vi "bin multiple xy graphs-b.vi"(2 "Error Bar Type":T1(ring), 3 "interval":dbl, 4 "FIXED X INTERVAL?":bool, 5 "parameter 2,3,4 vs 1":cluster{"y vector":dbl[], "avg optspec":dbl[]}[](graph)=[{"y vector"=array[1339 elements], "avg optspec"=array[1339 elements]}, {"y vector"=array[1339 elements], "avg optspec"=array[1339 elements]}, {"y vector"=array[1339 elements], "avg optspec"=array[1339 elements]}]) -> (0 "avgs and errors":dbl[][](array[numeric]), 1 "Array":cluster{"y vector":dbl[], "avg optspec":dbl[]}[](array[cluster]))   [LabVIEW 2009]
panel:
  out "xy graph":cluster{dbl[], dbl[]}[](graph)=[{[5.5, 15.5, 25.5, 35.5, 45.5, 55.5, 0.0], [0.1, 0.1, 0.15, 0.15, 0.2, 0.2, 0.0]}, {[5.5, 5.5, nan, 15.5, 15.5, nan, 25.5, 25.5, nan, 35.5, 35.5, nan, 45.5, 45.5, nan, 55.5, 55.5, nan, 0.0, 0.0, nan], [0.1, 0.1, nan, 0.1, 0.1, nan, 0.15, 0.15, nan, 0.15, 0.15, nan, 0.2, 0.2, nan, 0.2, 0.2, nan, 0.0, 0.0, nan]}, {[5.5, 15.5, 25.5, 35.5, 45.5, 55.5, 0.0], [5.5, 15.5, 25.5, 35.5, 45.5, 55.5, 0.0]}, {[5.5, 5.5, nan, 15.5, 15.5, nan, 25.5, 25.5, nan, 35.5, 35.5, nan, 45.5, 45.5, nan, 55.5, 55.5, nan, 0.0, 0.0, nan], [3.0, 8.0, nan, 13.0, 18.0, nan, 23.0, 28.0, nan, 33.0, 38.0, nan, 43.0, 48.0, nan, 53.0, 58.0, nan, 0.0, 0.0, nan]}]
  out "Array avgs and errors":dbl[][][](array[numeric])
  out "parameter 2,3,4 vs 2":cluster{"y vector":dbl[], "avg optspec":dbl[]}(graph)
  # "avgx\navgy\nerrorlow\nerrorhigh"
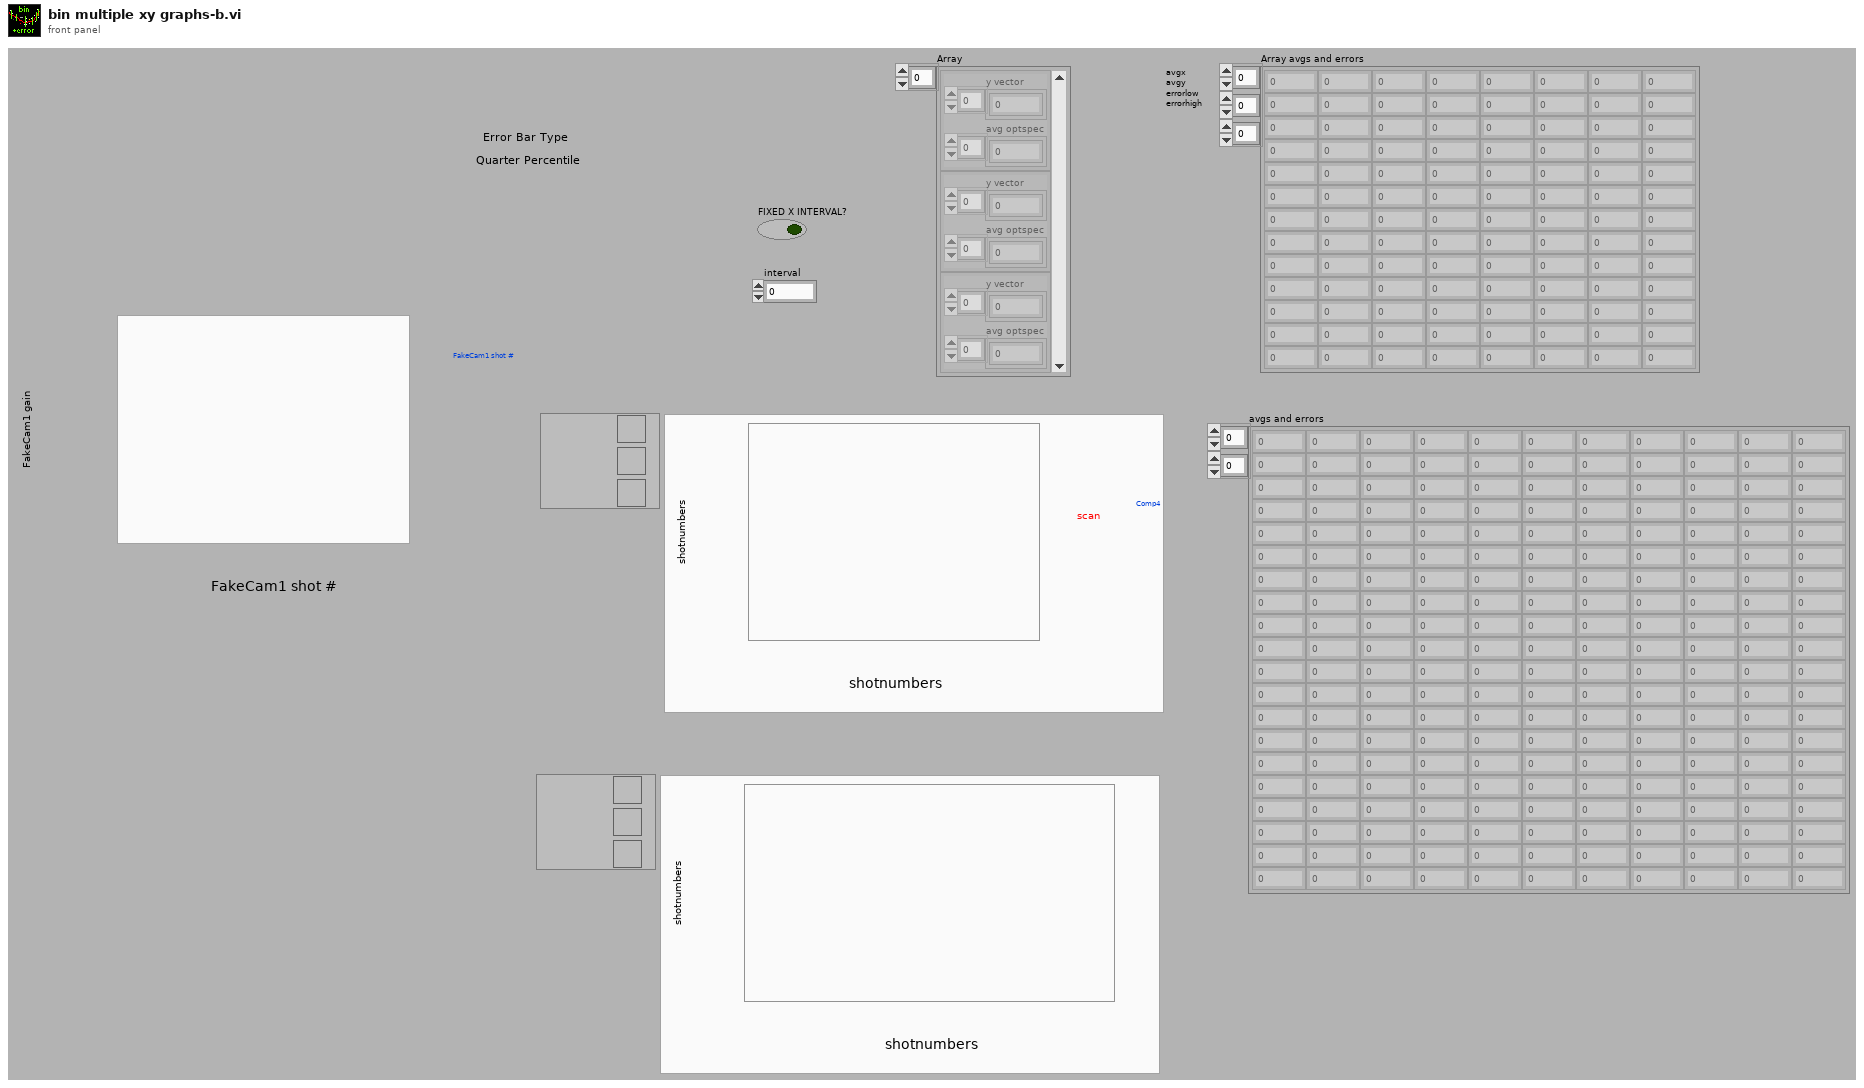
[diagram p1: front panel]
types:
  T1 = enum16{"Quarter Percentile", "Standard Deviation"}
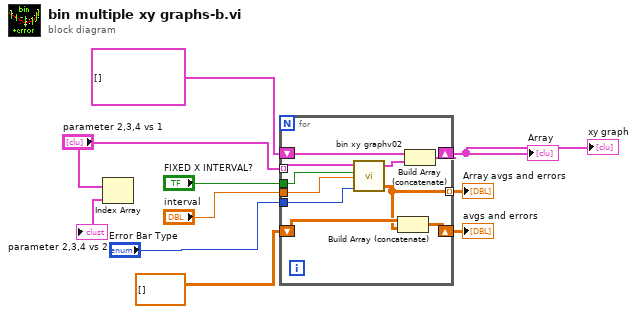
[diagram p0: block diagram]
diagram:
  n1 = Index Array(array="parameter 2,3,4 vs 1") -> (element=→"parameter 2,3,4 vs 2":cluster{"y vector":dbl[], "avg optspec":dbl[]})  [unwired: 1 in]
  n2 = for {
    tunnel: "parameter 2,3,4 vs 1" -> [w20] mode=indexing
    shift-right: [w17] -> w1
    shift-left: cluster{"y vector":dbl[], "avg optspec":dbl[]}[] [] -> [w19]
    tunnel: "FIXED X INTERVAL?" -> [w16]
    tunnel: "interval" -> [w15]
    tunnel: "Error Bar Type" -> [w14]
    shift-right: [w13] -> w7
    shift-left: dbl[][] [] -> [w12]
    tunnel: [w11] -> w3 mode=indexing
    n3 = call "bin xy graphv02.vi"("Error Bar Type"=w14, "interval"=w15, "FIXED X INTERVAL?"=w16, "Input Graph"=w20) -> ("Array avgs and errors"=w11:dbl[][], "Binned graph"=w18:cluster{"y vector":dbl[], "avg optspec":dbl[]}[])  [unwired: 1 out]
    n4 = Build Array (concatenate)(w12, w11) -> (w13:dbl[][])
    n5 = Build Array (concatenate)(w19, w18) -> (w17:cluster{"y vector":dbl[], "avg optspec":dbl[]}[])
  }
  "Array" <- w1
  "avgs and errors" <- w7
  "Array avgs and errors" <- w3
  "xy graph" <- w1
